vi "cached_threshold_read.vi"() -> ()   [LabVIEW 2018]
uses:
  <vilib>/rvi/Memory/Memory_Emulation/nirvimemoryFastEmulation.vi
  <vilib>/rvi/Memory/Memory_Emulation/nirvimemoryEmulation.vi
  <vilib>/rvi/Emulation/niFpgaEmulationIsFPGAContextNoSignature.vi
  <vilib>/rvi/DataTransferAndStorage/Container/Common/niFpgaContainerGetUniqueNameForEmu.vi
  <vilib>/rvi/Emulation/niFpgaProcessEmulError.vi
  <vilib>/rvi/Emulation/niFpgaSctlEmulationGetInTimedLoop.vi
  <vilib>/rvi/errors/nirviReportUnexpectedCaseInternalError (U32).vi
  <vilib>/rvi/DataTransferAndStorage/Container/XNode/niFpgaContainer.xnode
panel:
  out "value":fxp<+/-,32,16>
  in  "refresh":bool
  in  "index":u8
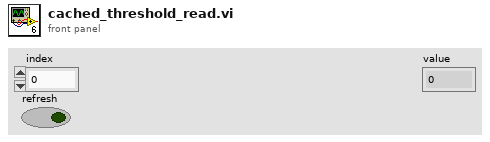
[diagram p1: front panel]
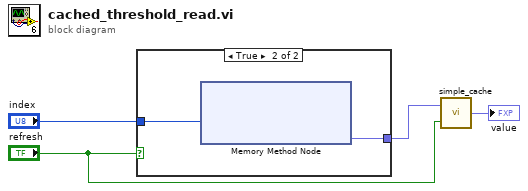
[diagram p0: block diagram]
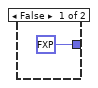
[diagram p2: hidden frame]
diagram:
  n1 = case shown="True" "refresh" {
    tunnel: [fxp<+/-,1,0> 0.0 ("Data") w7] -> w4
    tunnel: "index" -> [_ w6]
    frame False {
    }
    frame True {
      n2 = xnode ("Memory Method Node")("Address"=w6) -> ("Data"=w7:fxp<+/-,32,16>)  [unwired: 1 in, 1 out]
    }
  }
  n3 = call "simple_cache.vi"("refresh"="refresh", "new_val"=w4) -> ("$_val"=→"value":fxp<+/-,32,16>)
